vi "Set Waveform Chart Plot Values.vi"(8 "error in (no error)":errorcluster, 9 "Values":dbl[][](array[numeric]), 11 "WaveformChart in":refnum<vi>) -> (0 "error out":errorcluster, 3 "WaveformChart out":refnum<vi>)   [LabVIEW 2018]
doc: "Sets the values of plots in a waveform chart. Currently only supports waveform charts with a 2D numeric double data type."
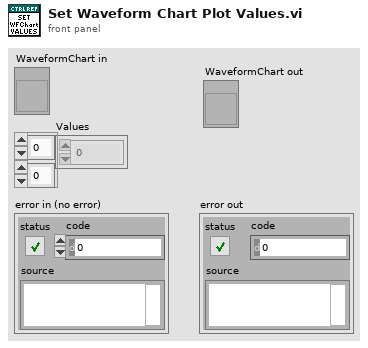
[diagram p1: front panel]
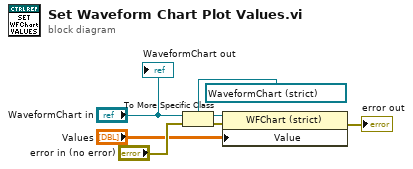
[diagram p0: block diagram]
diagram:
  n1 = To More Specific Class(target class=refnum<vi> refnum ("Waveform Chart"), reference="WaveformChart in", error in="error in (no error)") -> (specific class reference=w3:refnum<vi>, error out=w4:errorcluster)
  n2 = property on="Property Node" class="WFChart (strict)"(reference=w3, error in=w4, "Value"="Values") -> (error out=→"error out":errorcluster)  [unwired: 1 out]
  "WaveformChart out" <- "WaveformChart in"
